vi "Create_AO_WF.vi"(8 "error in":errorcluster) -> (0 "error out":errorcluster)   [LabVIEW 2025]
panel:
  out "Illumination analog waveforms":waveform(dbl)[](graph) caption="Output Waveform"
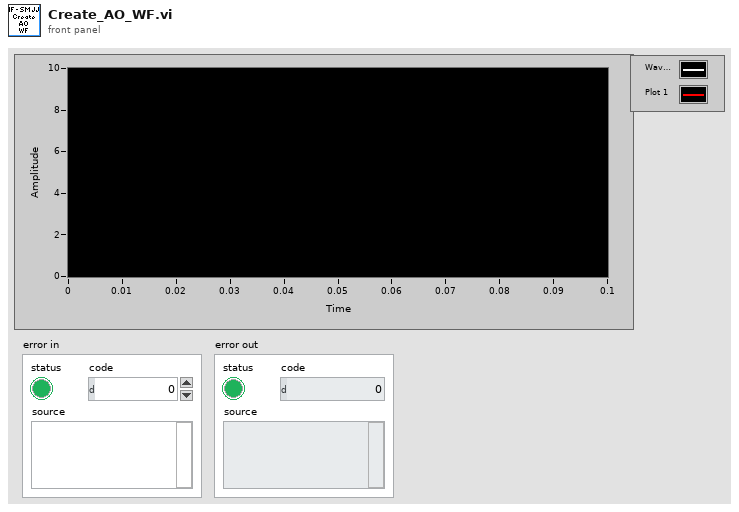
[diagram p1: front panel]
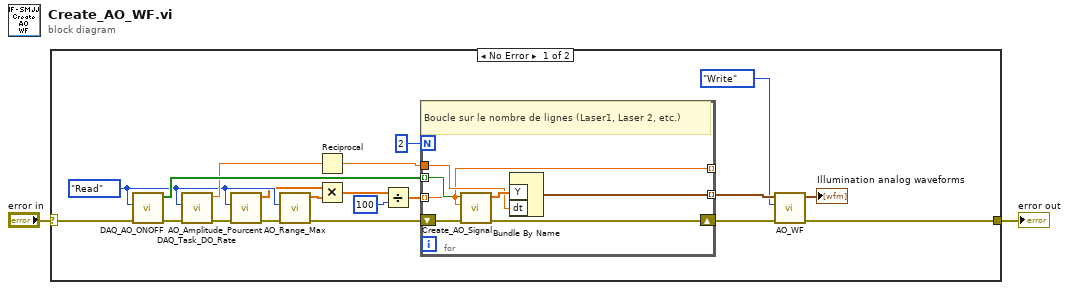
[diagram p0: block diagram]
diagram:
  n1 = case shown="No Error" "error in" {
    selector: "error in" -> [w22 w30]
    tunnel: [w20 w30] -> w1
    frame No Error {
      w9 = enum16{"Init", "Write", "Read"}."Read" ("Action")
      n2 = call "DAQ_AO_ONOFF.vi"("error in"=w22, "Action"=w9) -> ("error out"=w17:errorcluster, "AO | ON/OFF"=w19:bool[])  [unwired: 8 in]
      n3 = call "DAQ_Task_DO_Rate.vi"("error in"=w17, "Action"=w9) -> ("error out"=w13:errorcluster, "DO_Rate"=w16:dbl)  [unwired: 8 in]
      n4 = call "AO_Amplitude_Pourcent.vi"("error in"=w13, "Action"=w9) -> ("error out"=w12:errorcluster, "AO | %"=w6:dbl[])  [unwired: 8 in]
      n5 = call "AO_Range_Max.vi"("error in"=w12, "Action"=w9) -> ("error out"=w10:errorcluster, "AO | Max"=w5:dbl[])  [unwired: 8 in]
      n6 = Reciprocal(x=w16) -> (1/x=w14:dbl)
      n7 = Multiply(x=w6, y=w5) -> (x*y=w4:dbl[])
      n8 = Divide(x=w4, y=100) -> (x/y=w11:dbl[])
      n9 = for {
        N: 2 -> [_]
        shift-right: [w24] -> w21
        shift-left: w10 -> [w29]
        tunnel: w19 -> [w28] mode=indexing
        tunnel: w14 -> [w26]
        tunnel: [w25] -> w15 mode=indexing
        tunnel: [w23] -> _ mode=indexing
        tunnel: w11 -> [w23] mode=indexing
        # "Boucle sur le nombre de lignes (Laser1, Laser 2, etc.)"
        n10 = call "Create_AO_Signal.vi"("error in"=w29, "AO Amplitude"=w23, "ON / OFF"=w28) -> ("error out"=w24:errorcluster, "WF"=w27:dbl[])  [unwired: 7 in]
        n11 = Bundle By Name("Y"=w27, "dt"=w26) -> (w25:waveform(dbl))  [unwired: 1 in]
      }
      n12 = call "AO_WF.vi"("error in"=w21, "Action"=enum16{"Init", "Write", "Read"}."Write", "AO WF"=w15) -> ("error out"=w20:errorcluster, "AO WF"=→"Illumination analog waveforms":waveform(dbl)[])  [unwired: 7 in]
    }
    frame Error {
    }
  }
  "error out" <- w1
